vi "writeCRC.vi"(8 "error in (no error)":errorcluster, 10 "Length":i32, 11 "ModbusBuffer in":refnum<class "ModbusBufferBuilder.lvclass">) -> (0 "error out":errorcluster, 3 "ModbusBuffer out":refnum<class "ModbusBufferBuilder.lvclass">)   [LabVIEW 2016, in "ModbusBufferBuilder.lvclass"]
uses:
  ModbusBufferBuilder.lvclass
  ModbusBufferBuilder.lvclass/ModbusBufferBuilder.ctl
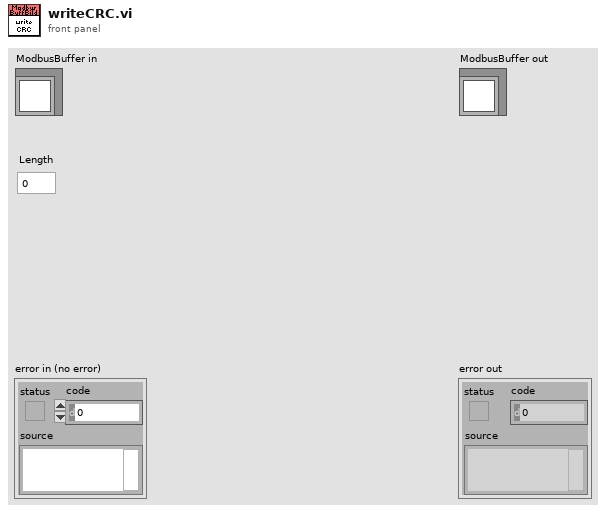
[diagram p1: front panel]
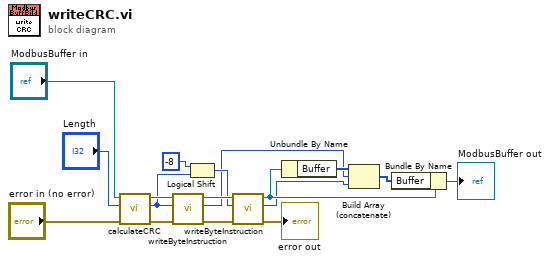
[diagram p0: block diagram]
diagram:
  n1 = call "calculateCRC.vi"("error in (no error)"="error in (no error)", "Length"="Length", "ModbusBuffer in"="ModbusBuffer in") -> ("error out"=w7:errorcluster, "CRC"=w5:u16, "ModbusBuffer out"=w9:refnum<class "ModbusBufferBuilder.lvclass">)  [unwired: 6 in]
  n2 = call "writeByteInstruction.vi"("error in (no error)"=w7, "Input"=w5, "ModbusBuffer in"=w9) -> ("error out"=w14:errorcluster, "Output"=w3:u16, "ModbusBuffer out"=w16:refnum<class "ModbusBufferBuilder.lvclass">)  [unwired: 6 in]
  n3 = Logical Shift(y=i16 -8, x=w5) -> (x << y=w15:u16)
  n4 = call "writeByteInstruction.vi"("error in (no error)"=w14, "Input"=w15, "ModbusBuffer in"=w16) -> ("error out"=→"error out":errorcluster, "Output"=w2:u16, "ModbusBuffer out"=w13:refnum<class "ModbusBufferBuilder.lvclass">)  [unwired: 6 in]
  n5 = Unbundle By Name(w13) -> ("Buffer"=w4:u16[])
  n6 = Build Array (concatenate)(w4, w3, w2) -> (w1:u16[])
  n7 = Bundle By Name(cluster=w13, "Buffer"=w1) -> (→"ModbusBuffer out":refnum<class "ModbusBufferBuilder.lvclass">)
